vi "DSF.Engine.Transceiver.Rx.vi"(8 "error in (no error)":errorcluster, 10 "Transfer Group in":refnum<class "DSF.Engine.Transfer Group.lvclass">, 11 "PXImc Transceiver in":refnum<class "DSF.Transceiver.PXImc.lvclass">) -> (0 "error out":errorcluster, 2 "Transfer Group out":refnum<class "DSF.Engine.Transfer Group.lvclass">, 3 "PXImc Transceiver out":refnum<class "DSF.Transceiver.PXImc.lvclass">)   [LabVIEW 2017, in "DSF.Transceiver.PXImc.lvlib" / "DSF.Transceiver.PXImc.lvclass"]
uses:
  DSF.Transceiver.PXImc.lvclass
  DSF Core/Built/Engine/DSF.Engine.lvlibp/Engine/Classes/Transfer/DSF.Engine.Transfer Group.lvclass
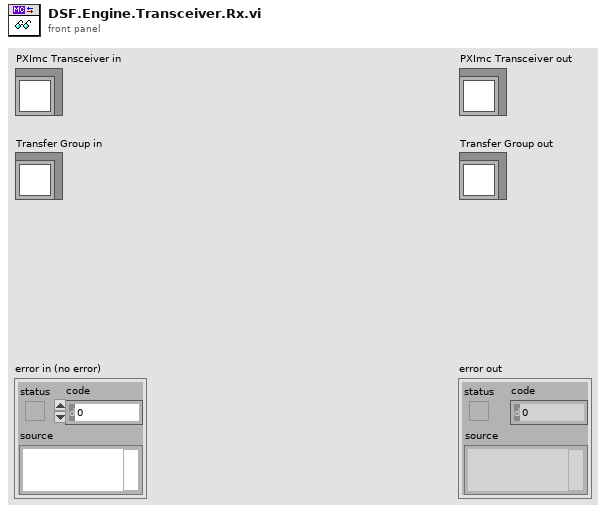
[diagram p1: front panel]
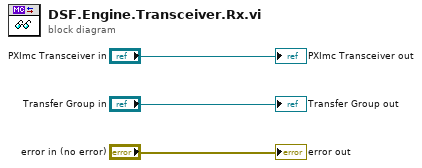
[diagram p0: block diagram]
diagram:
  "error out" <- "error in (no error)"
  "PXImc Transceiver out" <- "PXImc Transceiver in"
  "Transfer Group out" <- "Transfer Group in"
